vi "helper - polar plot grids.vi"(5 "[user-specified font]":T2, 7 "desired font(Application)":T4(ring)=enum."Application Font", 9 "polar attributes":T3 {"minimum" format="%0.2f"; "maximum" format="%0.2f"}, 10 "rect":T5={"left"=0, "top"=0, "right"=160, "bottom"=131}, 11 "picture":picture) -> (1 "grid measurements":T1 {"end angle" format="%0.2f"; "start angle" format="%0.2f"; "scale factors"."b" format="%0.2f"; "scale factors"."a" format="%0.2f"}, 3 "new picture":picture)   [LabVIEW 2011]
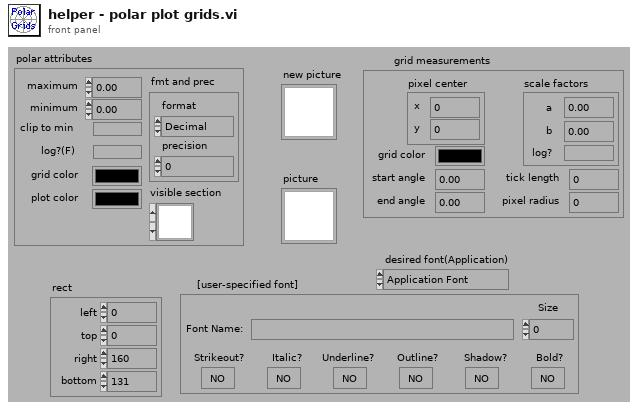
[diagram p1: front panel]
types:
  T1 = cluster{"pixel center":cluster{"x":i16, "y":i16}, "scale factors":cluster{"a":dbl, "b":dbl, "log?":bool}, "grid color":u32, "start angle":dbl, "end angle":dbl, "tick length":i16, "pixel radius":i32}
  T2 = cluster{"Font Name:":string, "Size":i16, "Strikeout?":bool, "Italic?":bool, "Underline?":bool, "Outline?":bool, "Shadow?":bool, "Bold?":bool}
  T3 = cluster{"maximum":dbl, "minimum":dbl, "clip to min":bool, "log?(F)":bool, "grid color":u32, "plot color":u32, "fmt and prec":cluster{"format":enum8{"Decimal", "Scientific", "Engineering", "Binary", "Octal", "Hex"}, "precision":u8}, "visible section":u16}
  T4 = enum16{"User-specified Font", "Application Font", "System Font", "Dialog Font"}
  T5 = cluster{"left":i16, "top":i16, "right":i16, "bottom":i16}
  T6 = cluster{"pixel center":cluster{"x":i16, "y":i16}, "scale factors":cluster{"a":dbl, "b":dbl, "log?(F)":bool}, "grid color":u32, "start angle":dbl, "end angle":dbl, "tick length":i16, "pixel radius":i32}
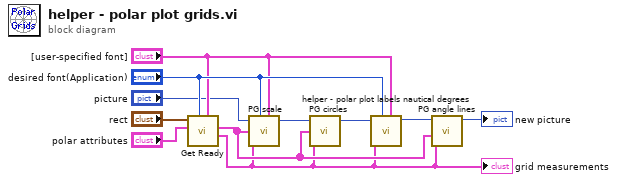
[diagram p0: block diagram]
diagram:
  n1 = call <vilib>:"Get Ready.vi"("polar attributes"="polar attributes", "rect"="rect", "desired font(Application)"="desired font(Application)", "[user-specified font]"="[user-specified font]") -> ("grid measurements"=w1:T6, "decade specs"=w7:cluster{"radius":i16, "label":string}[])  [unwired: 6 in]
  "grid measurements" <- w1
  n2 = call <vilib>:"PG scale.vi"("picture"="picture", "desired font(Application)"="desired font(Application)", "decade specs"=w7, "grid measurements"=w1, "[user-specified font]"="[user-specified font]") -> ("new picture"=w11:picture)  [unwired: 4 in]
  n3 = call <vilib>:"PG circles.vi"("picture"=w11, "decade specs"=w7, "grid measurements"=w1) -> ("new picture"=w10:picture)  [unwired: 6 in]
  n4 = call "helper - polar plot labels nautical degrees.vi"("grid measurements"=w1, "picture"=w10, "desired font(Application)"="desired font(Application)", "[user-specified font]"="[user-specified font]") -> ("new picture"=w9:picture)  [unwired: 3 in]
  n5 = call <vilib>:"PG angle lines.vi"("grid measurements"=w1, "decade specs"=w7, "picture"=w9) -> ("new picture"=→"new picture":picture)  [unwired: 8 in]
